vi "Set Scan Values.vi"(7 "No. of steps":u32, 8 "error in (no error)":errorcluster, 9 "Array from List":T1[](array[typedef]), 10 "Array of Parameters":T2[](array[typedef]), 11 "Scan SBlock in":refnum<class "Scan SBlock.lvclass">) -> (0 "error out":errorcluster, 3 "Scan SBlock out":refnum<class "Scan SBlock.lvclass">)   [LabVIEW 2020, in "TALOS.lvlib" / "Run Utilities.lvlib" / "Scan SBlock.lvclass"]
doc: "Create a new Schedule Block Object with specified Advanced Panel Controls Values"
uses:
  Scan SBlock.lvclass
  Advanced Parameters.ctl
  Advanced Panel Parameter Mode.ctl
  Advanced Parameters - list.ctl
  Scan SBlock.lvclass/Scan SBlock.ctl
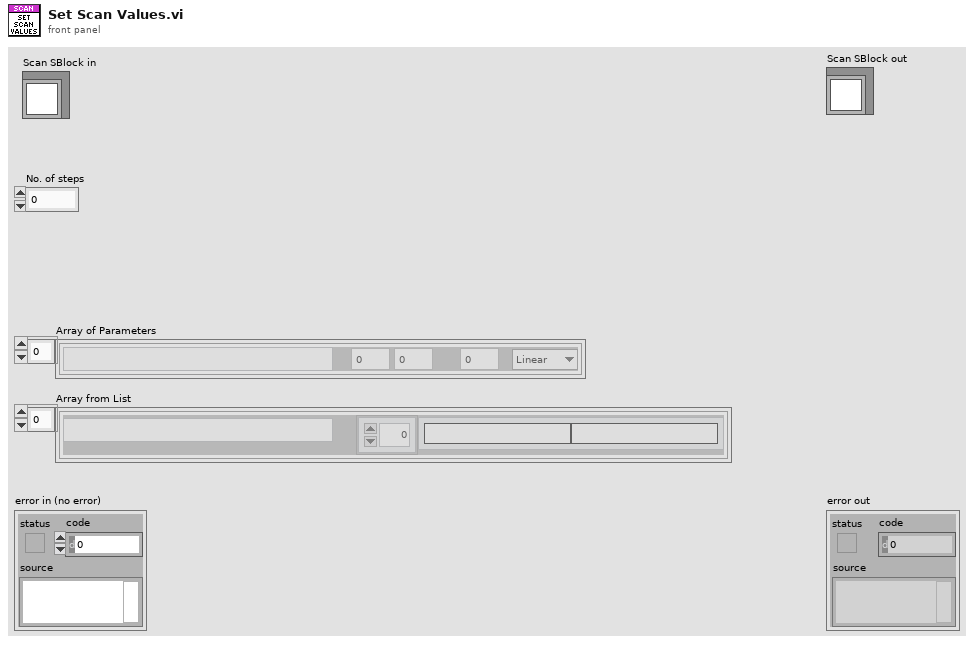
[diagram p1: front panel]
types:
  T1 = typedef "TALOS.lvlib/Run Utilities.lvlib/Scan SBlock.lvclass/Advanced Parameters - list.ctl" = cluster{"Param":string, "List of values":string[]}
  T2 = typedef "TALOS.lvlib/Run Utilities.lvlib/Scan SBlock.lvclass/Advanced Parameters.ctl" = cluster{"Param":string, "From":dbl, "To":dbl, "Step":dbl, "Mode":T3}
  T3 = typedef "TALOS.lvlib/Run Utilities.lvlib/Scan SBlock.lvclass/Advanced Panel Parameter Mode.ctl" = enum16{"Linear", "Log", "LINKED"}
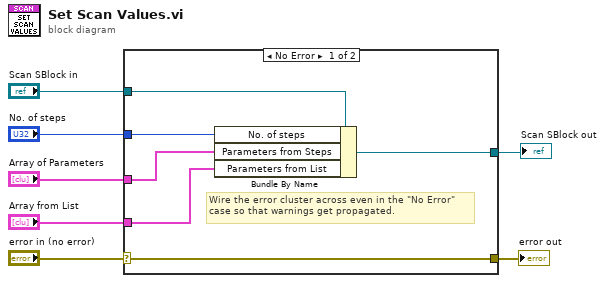
[diagram p0: block diagram]
diagram:
  n1 = case shown="No Error" "error in (no error)" {
    selector: "error in (no error)" -> [w13 w15]
    tunnel: [w13 w15] -> w6
    tunnel: [w12 w14] -> w2
    tunnel: "No. of steps" -> [w11 _]
    tunnel: "Array of Parameters" -> [w10 _]
    tunnel: "Array from List" -> [w9 _]
    tunnel: "Scan SBlock in" -> [w8 w14]
    frame No Error {
      # "Wire the error cluster across even in the \"No Error\"\ncase so that warnings get propagated."
      n2 = Bundle By Name(cluster=w8, "No. of steps"=w11, "Parameters from Steps"=w10, "Parameters from List"=w9) -> (w12:refnum<class "Scan SBlock.lvclass">)
    }
    frame Error {
    }
  }
  "error out" <- w6
  "Scan SBlock out" <- w2
